vi "Close shutter on MC stop.vi"(8 "error in (no error)":errorcluster) -> (0 "error out":errorcluster)   [LabVIEW 2020]
uses:
  Typedefs/Shutter Function Enum.ctl
  Global Variables/General Globals.vi
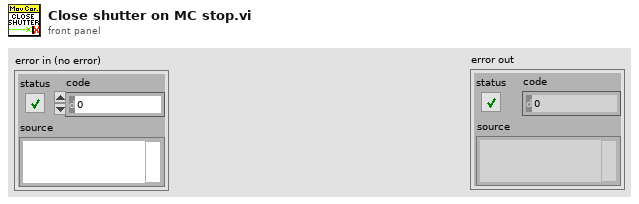
[diagram p1: front panel]
types:
  T1 = typedef "Shutter Function Enum.ctl" = enum16{"Open Shutter", "Close Shutter"}
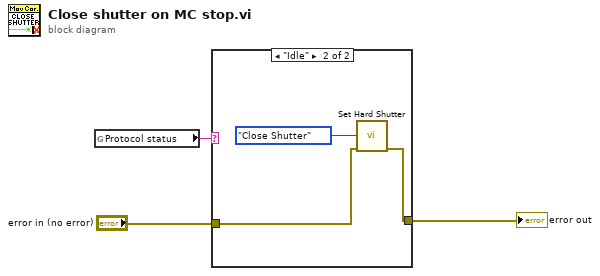
[diagram p0: block diagram]
diagram:
  n1 = global read "General Globals.vi" "Protocol status"() -> (w3:string)
  n2 = case shown="\"Idle\"" w3 {
    tunnel: "error in (no error)" -> [w4 w6]
    tunnel: [w4 w5] -> w1
    frame Default {
    }
    frame "Idle" {
      n3 = call "Set Hard Shutter.vi"("Error In"=w6, "Shutter Function"=Shutter_Function_Enum."Close Shutter") -> ("Error Out"=w5:errorcluster)  [unwired: 9 in]
    }
  }
  "error out" <- w1
